vi "手动打印功能.vi"(7 "日期时间记录":T1, 8 "错误输入（无错误）":errorcluster, 9 "流水号（3位）":string, 10 "班次":string, 11 "路径":path) -> (0 "error out":errorcluster caption="错误输出", 3 "Print":i32(ring) items=["btSuccess", "btTimeout", "btFailure"])   [LabVIEW 2018]
uses:
  <vilib>/Utility/miscctls.llb/LVDateTimeRec.ctl
panel:
  in  "BarTender.IBtApplication":refnum<k7>
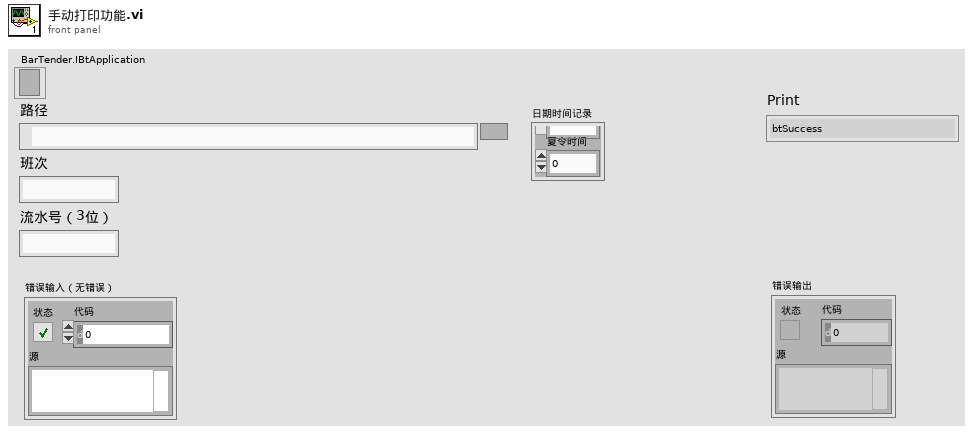
[diagram p1: front panel]
types:
  T1 = typedef "LVDateTimeRec.ctl" = cluster{"fractional second":dbl, "second":i32, "minute":i32, "hour":i32, "day of month":i32, "month":i32, "year":i32, "day of week":i32, "day of year":i32, "DST":i32}
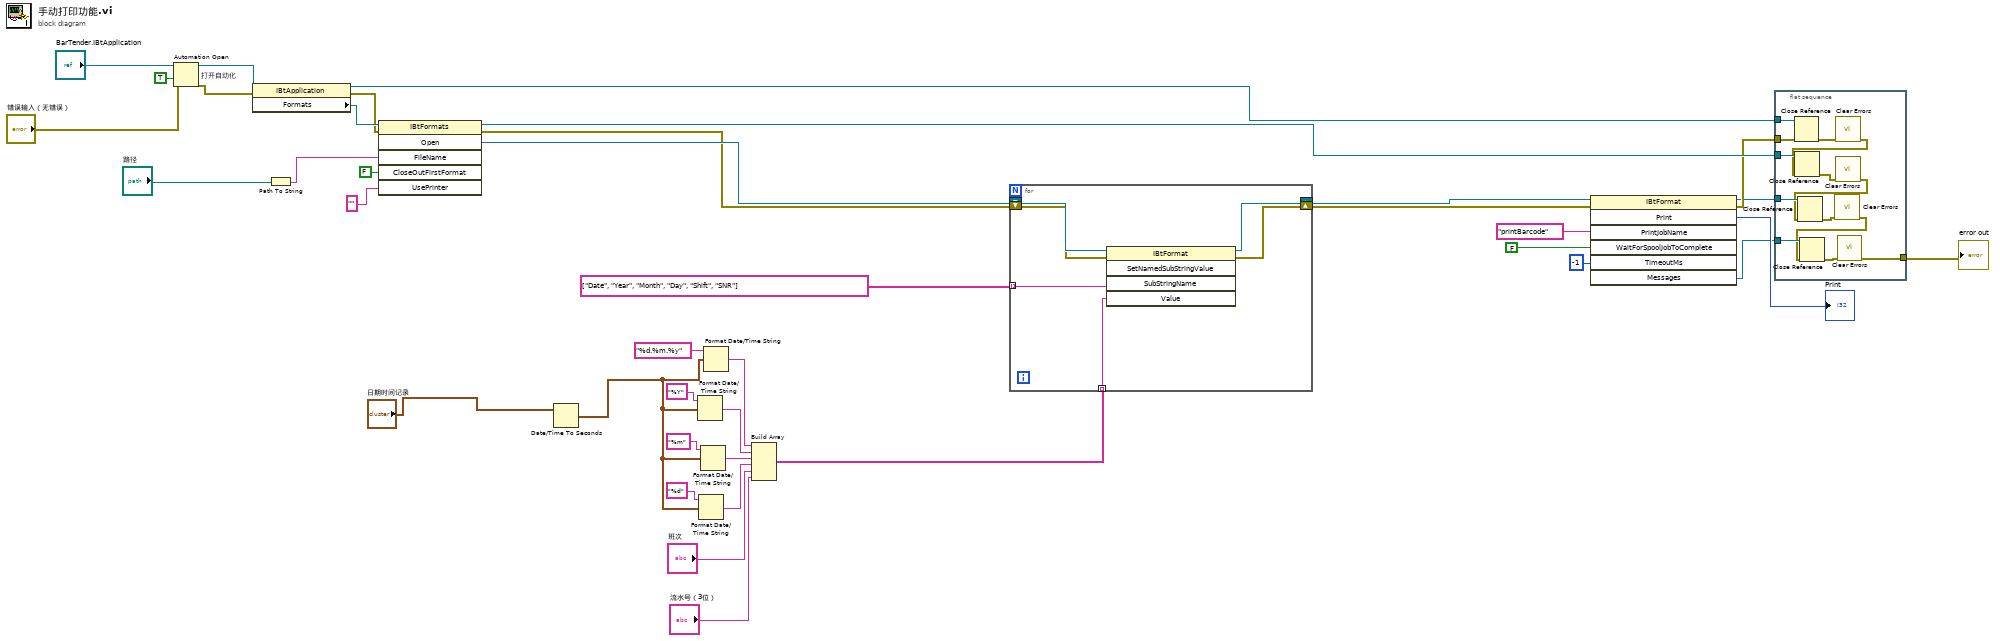
[diagram p0: block diagram]
diagram:
  n1 = Automation Open "打开自动化"(error in (no error)="错误输入（无错误）", Automation Refnum="BarTender.IBtApplication", 9:TRUE ("打开新实例（假）")) -> (Automation Refnum=w39:refnum<k7>, error out=w36:errorcluster)  [unwired: 1 in]
  n2 = property on="属性节点" class="IBtApplication"(reference=w39, error in=w36) -> (reference out=w34:refnum<k7>, error out=w35:errorcluster, "Formats"=w38:refnum<k7>)
  n3 = Path To String(path="路径") -> (string=w21:string)
  n4 = invoke on="调用节点" class="IBtFormats" method="Open"(reference=w38, error in=w35, "FileName"=w21, "CloseOutFirstFormat"=FALSE, "UsePrinter"="") -> (reference out=w33:refnum<k7>, error out=w22:errorcluster, "Open"=w23:refnum<k7>)  [unwired: 1 in, 3 out]
  n5 = Date/Time To Seconds(2:"日期时间记录") -> (0:w2:timestamp)  [unwired: 1 in]
  n6 = Format Date/Time String(time format string (%c)="%Y" ("时间格式字符串(%c)"), seconds (now)=w2) -> (date/time string=w9:string)  [unwired: 1 in]
  n7 = Format Date/Time String(time format string (%c)="%d" ("时间格式字符串(%c)"), seconds (now)=w2) -> (date/time string=w7:string)  [unwired: 1 in]
  n8 = Format Date/Time String(time format string (%c)="%m" ("时间格式字符串(%c)"), seconds (now)=w2) -> (date/time string=w8:string)  [unwired: 1 in]
  n9 = Format Date/Time String(time format string (%c)="%d.%m.%y" ("时间格式字符串(%c)"), seconds (now)=w2) -> (date/time string=w13:string)  [unwired: 1 in]
  n10 = Build Array(w13, w9, w8, w7, "班次", "流水号（3位）") -> (w12:string[])
  n11 = for {
    shift-right: [w43] -> w16
    shift-left: w23 -> [w45]
    shift-right: [w42] -> w15
    shift-left: w22 -> [w44]
    tunnel: string[] ["Date", "Year", "Month", "Day", "Shift", "SNR"] -> [w41] mode=indexing
    tunnel: w12 -> [w40] mode=indexing
    n12 = invoke on="调用节点" class="IBtFormat" method="SetNamedSubStringValue"(reference=w45, error in=w44, "SubStringName"=w41, "Value"=w40) -> (reference out=w43:refnum<k7>, error out=w42:errorcluster)  [unwired: 1 in, 3 out]
  }
  n13 = invoke on="调用节点" class="IBtFormat" method="Print"(reference=w16, error in=w15, "PrintJobName"="printBarcode", "WaitForSpoolJobToComplete"=FALSE, "TimeoutMs"=-1) -> (reference out=w26:refnum<k7>, error out=w27:errorcluster, "Print"=→"Print":i32, "Messages"=w17:refnum<k7>)  [unwired: 2 in, 3 out]
  n14 = flat-sequence {
    tunnel: w34 -> [w58]
    tunnel: w33 -> [w57]
    tunnel: w27 -> [w56]
    tunnel: w26 -> [w55]
    tunnel: w17 -> [w48]
    tunnel: [w46] -> w3
    frame #0 {
      n15 = Close Reference(reference=w58, error in (no error)=w56) -> (error out=w51:errorcluster)
      n16 = call <vilib>:"Clear Errors.vi"("error in (no error)"=w51) -> ("error out"=w50:errorcluster)  [unwired: 5 in, 1 out]
      n17 = Close Reference(reference=w57, error in (no error)=w50) -> (error out=w53:errorcluster)
      n18 = call <vilib>:"Clear Errors.vi"("error in (no error)"=w53) -> ("error out"=w52:errorcluster)  [unwired: 5 in, 1 out]
      n19 = Close Reference(reference=w55, error in (no error)=w52) -> (error out=w54:errorcluster)
      n20 = call <vilib>:"Clear Errors.vi"("error in (no error)"=w54) -> ("error out"=w47:errorcluster)  [unwired: 5 in, 1 out]
      n21 = Close Reference(reference=w48, error in (no error)=w47) -> (error out=w49:errorcluster)
      n22 = call <vilib>:"Clear Errors.vi"("error in (no error)"=w49) -> ("error out"=w46:errorcluster)  [unwired: 5 in, 1 out]
    }
  }
  "error out" <- w3
